vi "Set Motor Inertia.vi"(8 "error in (no error)":errorcluster, 10 "Motor Inertia":dbl, 11 "Link in":refnum<class "Link.lvclass">) -> (0 "error out":errorcluster, 3 "Link out":refnum<class "Link.lvclass">)   [LabVIEW 2013, in "Link.lvclass"]
uses:
  Link.lvclass
  Link.lvclass/Link.ctl
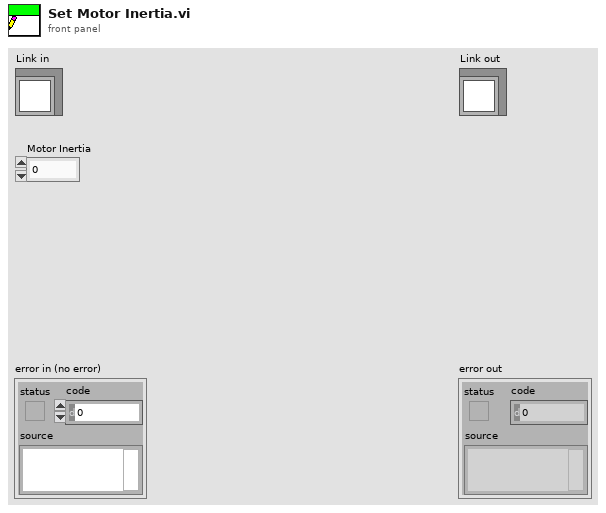
[diagram p1: front panel]
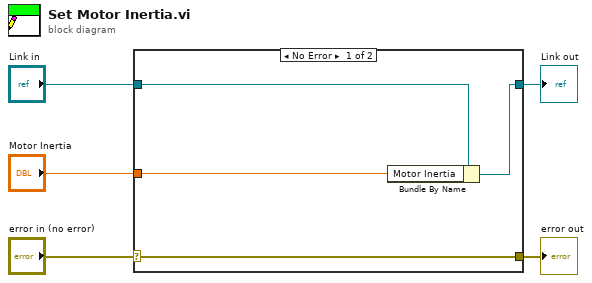
[diagram p0: block diagram]
diagram:
  n1 = case shown="No Error" "error in (no error)" {
    selector: "error in (no error)" -> [w9 w10]
    tunnel: [w9 w10] -> w4
    tunnel: [w7 w11] -> w2
    tunnel: "Link in" -> [w8 w11]
    tunnel: "Motor Inertia" -> [w6 _]
    frame No Error {
      n2 = Bundle By Name(cluster=w8, "Motor Inertia"=w6) -> (w7:refnum<class "Link.lvclass">)
    }
    frame Error {
    }
  }
  "error out" <- w4
  "Link out" <- w2
